vi "test config.vi"(8 "error in (no error)":errorcluster, 11 "Device position":string) -> (0 "error out":errorcluster)   [LabVIEW 2023]
uses:
  TDK20-38 API.lvlib
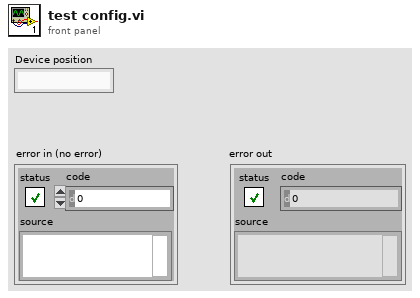
[diagram p1: front panel]
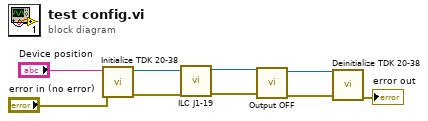
[diagram p0: block diagram]
diagram:
  n1 = call "Initialize TDK 20-38.vi"("error in (no error)"="error in (no error)", "Device position"="Device position") -> ("error out"=w6:errorcluster, "VISA out"=w7:refnum<visa-resource-name>)  [unwired: 8 in]
  n2 = call "ILC J1-19.vi"("error"=w6, "VISA"=w7) -> ("error out"=w4:errorcluster, "VISA out"=w5:refnum<visa-resource-name>)  [unwired: 8 in]
  n3 = call "Output OFF.vi"("error"=w4, "VISA"=w5) -> ("error out"=w2:errorcluster, "VISA out"=w3:refnum<visa-resource-name>)  [unwired: 8 in]
  n4 = call "Deinitialize TDK 20-38.vi"("error"=w2, "VISA name"=w3) -> ("error out"=→"error out":errorcluster)  [unwired: 9 in]
